vi "Przenies param rej szybka FVG.vi"(5 "Śledzenie In":enum16{"Obwiednia", "Migawka"}(ring), 7 "Czas In":i32, 8 "error in (no error)":errorcluster, 10 "Start In":bool, 11 "Akcja":T1) -> (0 "error out":errorcluster, 2 "Start Out":bool, 3 "Restart Out":bool, 4 "Śledzenie Out":enum16{"Obwiednia", "Migawka"}(ring), 6 "Czas Out":i32)   [LabVIEW 2013]
doc: "Przenosi parametry rejestracji szybkiej\noraz obsługuje reset okna rejestracji"
uses:
  Kontrolki/FVGs/FVG akwizycje akcje.ctl
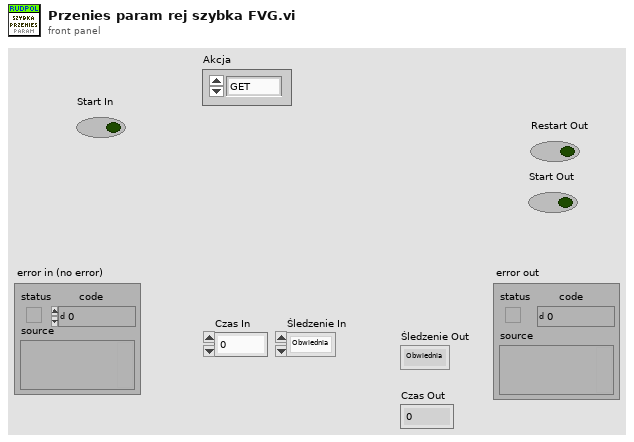
[diagram p1: front panel]
types:
  T1 = typedef "FVG akwizycje akcje.ctl" = enum16{"GET", "GETr", "SET"}
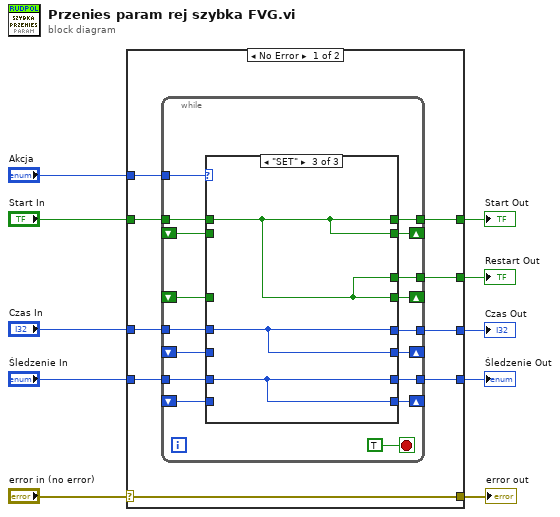
[diagram p0: block diagram]
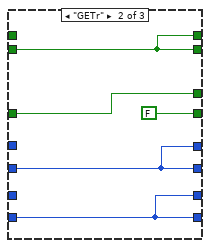
[diagram p3: hidden frame]
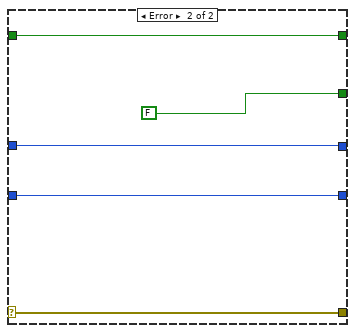
[diagram p4: hidden frame]
diagram:
  n1 = case shown="No Error" "error in (no error)" {
    selector: "error in (no error)" -> [w19 w53]
    tunnel: [w19 w53] -> w9
    tunnel: "Akcja" -> [w18 _]
    tunnel: "Start In" -> [w17 w51]
    tunnel: "Czas In" -> [w16 w50]
    tunnel: "Śledzenie In" -> [w15 w49]
    tunnel: [w14 w51] -> w3
    tunnel: [w11 FALSE ("Start In")] -> w4
    tunnel: [w13 w50] -> w2
    tunnel: [w12 w49] -> w1
    frame No Error {
      n2 = while {
        tunnel: w18 -> [w35]
        tunnel: w17 -> [w34]
        tunnel: w16 -> [w33]
        tunnel: w15 -> [w32]
        shift-right: [w31] -> _
        shift-left: _ -> [w30]
        shift-right: [w29] -> _
        shift-left: _ -> [w25]
        shift-right: [w28] -> _
        shift-left: _ -> [w24]
        shift-right: [w27] -> _
        shift-left: _ -> [w22]
        tunnel: [w26] -> w14
        tunnel: [w23] -> w13
        tunnel: [w21] -> w12
        tunnel: [w20] -> w11
        stop <- TRUE stop-if-true
        n3 = case shown="\"SET\"" w35 {
          tunnel: w34 -> [_ _ w46]
          tunnel: w33 -> [_ _ w47]
          tunnel: w32 -> [_ _ w48]
          tunnel: [w40 w43 w46] -> w31
          tunnel: w30 -> [w40 w43 _]
          tunnel: [w37 FALSE ("Start In") w46] -> w29
          tunnel: [w39 w45 w47] -> w28
          tunnel: [w38 w44 w48] -> w27
          tunnel: [w40 w43 w46] -> w26
          tunnel: w25 -> [w37 w41 _]
          tunnel: w24 -> [w39 w45 _]
          tunnel: [w39 w45 w47] -> w23
          tunnel: w22 -> [w38 w44 _]
          tunnel: [w38 w44 w48] -> w21
          tunnel: [w37 w41 w46] -> w20
          frame "GET", Default {
          }
          frame "GETr" {
          }
          frame "SET" {
          }
        }
      }
    }
    frame Error {
    }
  }
  "error out" <- w9
  "Restart Out" <- w4
  "Czas Out" <- w2
  "Śledzenie Out" <- w1
  "Start Out" <- w3
